vi "Example_analog_read.vi"() -> ()   [LabVIEW 2022 SP3]
uses:
  usbtmc_scpi_labtool.lvlib
panel:
  in  "ID Query (True)":bool=TRUE
  in  "ID query string":string="PICO-PI,LABTOOL"
  out "analog out":i32
  in  "Pin":u8 max=7 step=1
  in  "stop":bool
  in  "VISA resource name in":refnum<visa-resource-name>
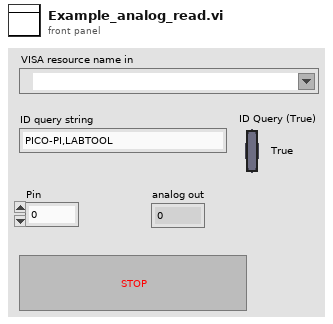
[diagram p1: front panel]
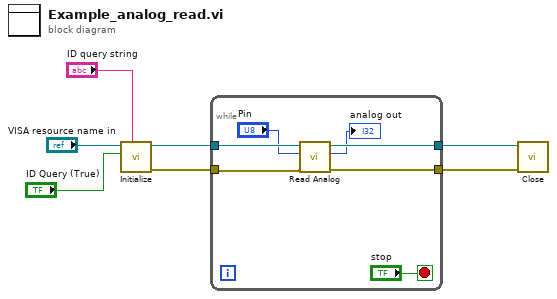
[diagram p0: block diagram]
diagram:
  n1 = call "Initialize.vi"("ID query string"="ID query string", "ID Query (True)"="ID Query (True)", "VISA resource name in"="VISA resource name in") -> ("error out"=w4:errorcluster, "VISA resource name out"=w5:refnum<visa-resource-name>)  [unwired: 7 in]
  n2 = while {
    tunnel: [w12] -> w6
    tunnel: w5 -> [w13]
    tunnel: w4 -> [w11]
    tunnel: [w10] -> w3
    stop <- "stop" stop-if-true
    n3 = call "Read Analog.vi"("error in (no error)"=w11, "Pin"="Pin", "VISA resource name"=w13) -> ("error out"=w10:errorcluster, "analog out"=→"analog out":i32, "VISA resource name out"=w12:refnum<visa-resource-name>)  [unwired: 6 in]
  }
  n4 = call "Close.vi"("error in (no error)"=w3, "VISA resource name"=w6) -> ()  [unwired: 10 in]
